vi "IsLogStopTriggered.vi"(7 "Application Configuration":T3={"DUT"={"Count"=1, "Wirings"=[], "Names"=[]}, "Log"={"Start"={"Trigger Type"=enum."Immediate", "Timer (sec)"=0.0, "Digital IO Line"=0, "Digital IO Edge"=enum."Rising"}, "Rollover"={"Trigger Type"=enum."None", "Timer (sec)"=0.0, "File Size (MB)"=0, "Digital IO Line"=0, "Digital IO Edge"=enum."Rising"}, "Stop"={"Trigger Type"=enum."None", "Timer (sec)"=0.0, "File Size (MB)"=0, "Digital IO Line"=0, "Digital IO Edge"=enum."Rising"}}, "Trigger"={"Input"={"Type"=enum."None", "Timeout (ms)"=0, "Delay (ms)"=0, "Digital IO Line (1-14)"=0, "Digital IO Mode"=enum."Falling"}, "Output"={"Type"=enum."None", "Delay (ms)"=0, "Digital IO Line (1-14)"=0, "Digital IO Mode"=enum."Falling", "Digital IO Pulse Width (sec)"=0.0}}, "Sources"=[], "Measures"=[]} {"Measures"."Count" min=1 step=1; "Trigger"."Output"."Digital IO Line (1-14)" min=1 max=14 step=1}, 8 "Error In":errorcluster, 11 "Log Data":T1[](array[typedef])) -> (0 "Error Out":errorcluster, 3 "Triggered?":bool)   [LabVIEW 2013]
uses:
  Setup.ctl
  DUTConfiguration.ctl
  driver/Public/Controls/SMUSense.ctl
  LogConfiguration.ctl
  LogStartConfiguration.ctl
  LogStartTriggerType.ctl
  LogDigitalIOTriggerEdge.ctl
  LogRolloverConfiguration.ctl
  LogRolloverTriggerType.ctl
  LogStopConfiguration.ctl
  LogStopTriggerType.ctl
  TriggerConfiguration.ctl
  TriggerInputConfiguration.ctl
  TriggerInputType.ctl
  driver/Public/Controls/TriggerMode.ctl
  TriggerOutputConfiguration.ctl
  TriggerOutputType.ctl
  SourceConfiguration.ctl
  SourceFunction.ctl
  MeasureConfiguration.ctl
  HardwareLogData.ctl
  HardwareDisplayData.ctl
  driver/Keithley-2602.lvlib
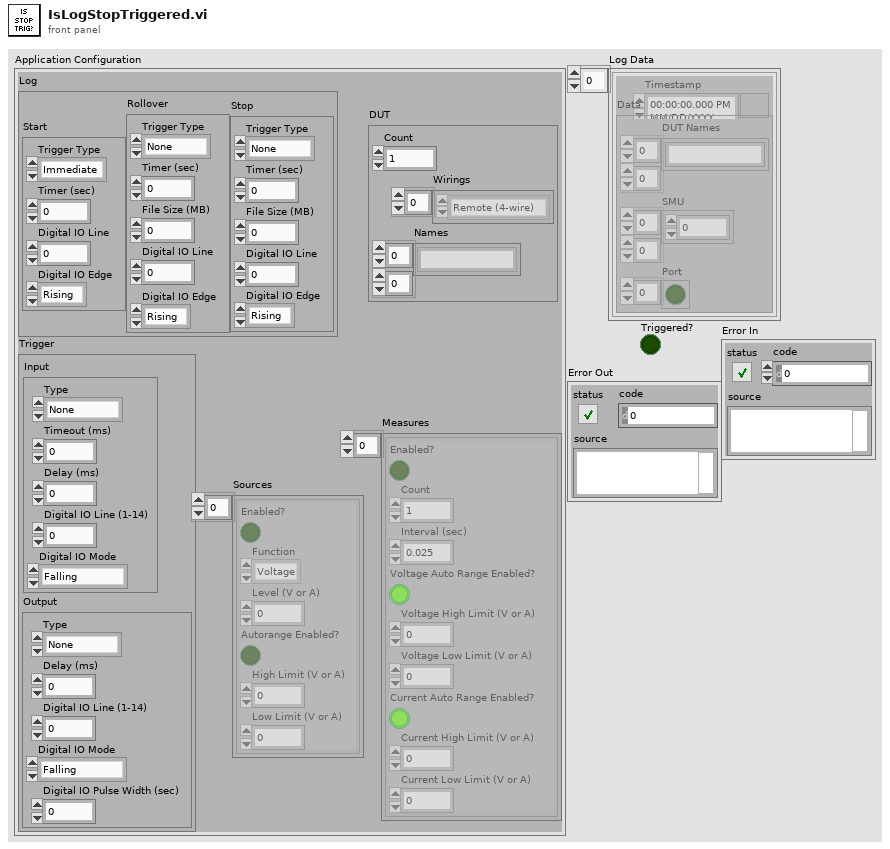
[diagram p1: front panel]
types:
  T1 = typedef "HardwareLogData.ctl" = cluster{"Timestamp":timestamp, "Data":T2}
  T2 = typedef "HardwareDisplayData.ctl" = cluster{"DUT Names":string[][], "SMU":dbl[][], "Port":bool[]}
  T3 = typedef "Setup.ctl" = cluster{"DUT":T4, "Log":T6, "Trigger":T14, "Sources":T20[], "Measures":T22[]}
  T4 = typedef "DUTConfiguration.ctl" = cluster{"Count":u32, "Wirings":T5[], "Names":string[][]}
  T5 = typedef "Keithley-2602.lvlib/SMUSense.ctl" = enum16{"Local (2-wire)", "Remote (4-wire)", "Calibration"}
  T6 = typedef "LogConfiguration.ctl" = cluster{"Start":T7, "Rollover":T10, "Stop":T12}
  T7 = typedef "LogStartConfiguration.ctl" = cluster{"Trigger Type":T8, "Timer (sec)":dbl, "Digital IO Line":u8, "Digital IO Edge":T9}
  T8 = typedef "LogStartTriggerType.ctl" = enum16{"Immediate", "User", "Timer", "Digital IO"}
  T9 = typedef "LogDigitalIOTriggerEdge.ctl" = enum16{"Rising", "Falling"}
  T10 = typedef "LogRolloverConfiguration.ctl" = cluster{"Trigger Type":T11, "Timer (sec)":dbl, "File Size (MB)":u32, "Digital IO Line":u8, "Digital IO Edge":T9}
  T11 = typedef "LogRolloverTriggerType.ctl" = enum16{"None", "Timer", "File Size", "Digital IO"}
  T12 = typedef "LogStopConfiguration.ctl" = cluster{"Trigger Type":T13, "Timer (sec)":dbl, "File Size (MB)":u32, "Digital IO Line":u8, "Digital IO Edge":T9}
  T13 = typedef "LogStopTriggerType.ctl" = enum16{"None", "User", "Timer", "File Size", "Digital IO"}
  T14 = typedef "TriggerConfiguration.ctl" = cluster{"Input":T15, "Output":T18}
  T15 = typedef "TriggerInputConfiguration.ctl" = cluster{"Type":T16, "Timeout (ms)":u32, "Delay (ms)":u32, "Digital IO Line (1-14)":u8, "Digital IO Mode":T17}
  T16 = typedef "TriggerInputType.ctl" = enum16{"None", "Digital IO", "Bus"}
  T17 = typedef "Keithley-2602.lvlib/TriggerMode.ctl" = enum16{"Falling", "Rising", "Either", "Synchronous"}
  T18 = typedef "TriggerOutputConfiguration.ctl" = cluster{"Type":T19, "Delay (ms)":u32, "Digital IO Line (1-14)":u8, "Digital IO Mode":T17, "Digital IO Pulse Width (sec)":dbl}
  T19 = typedef "TriggerOutputType.ctl" = enum16{"None", "Digital IO", "Bus"}
  T20 = typedef "SourceConfiguration.ctl" = cluster{"Enabled?":bool, "Function":T21, "Level (V or A)":dbl, "Autorange Enabled?":bool, "High Limit (V or A)":dbl, "Low Limit (V or A)":dbl}
  T21 = typedef "SourceFunction.ctl" = enum16{"Voltage", "Current"}
  T22 = typedef "MeasureConfiguration.ctl" = cluster{"Enabled?":bool, "Count":u8, "Interval (sec)":dbl, "Voltage Auto Range Enabled?":bool, "Voltage High Limit (V or A)":dbl, "Voltage Low Limit (V or A)":dbl, "Current Auto Range Enabled?":bool, "Current High Limit (V or A)":dbl, "Current Low Limit (V or A)":dbl}
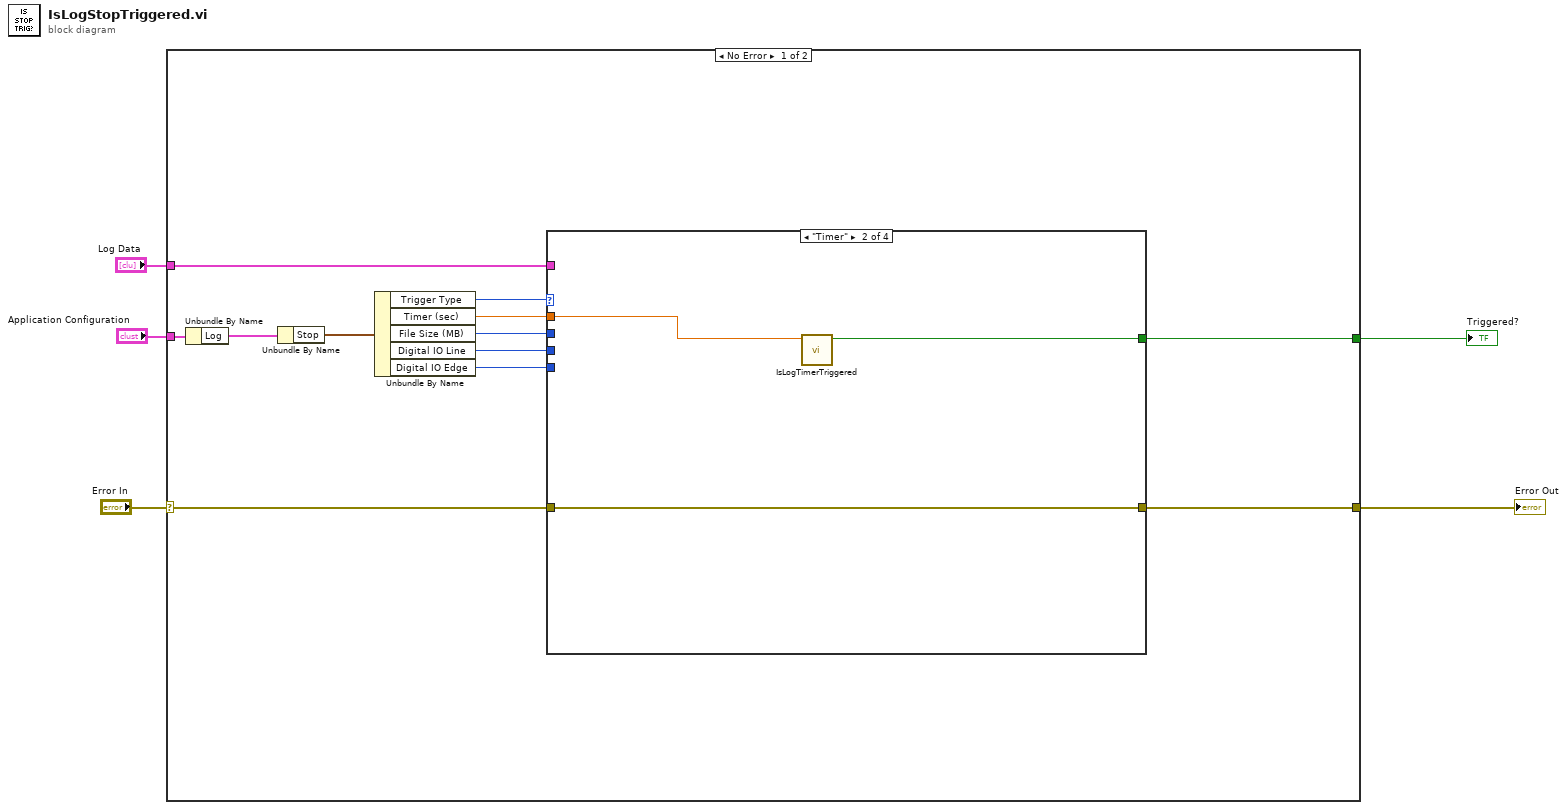
[diagram p0: block diagram]
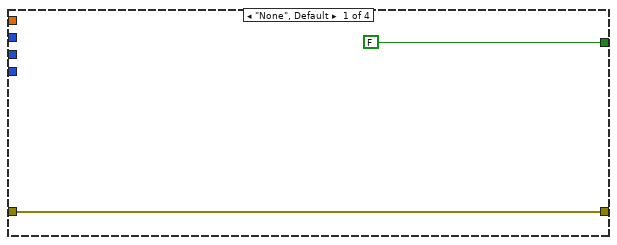
[diagram p2: hidden frame]
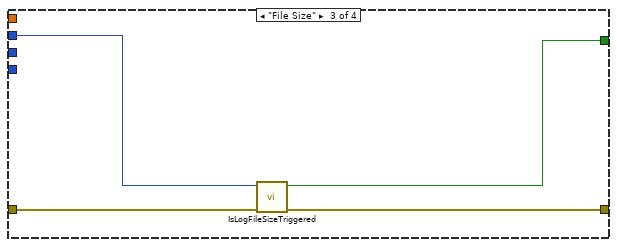
[diagram p3: hidden frame]
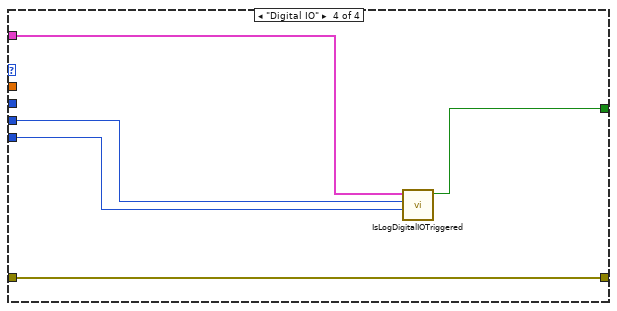
[diagram p4: hidden frame]
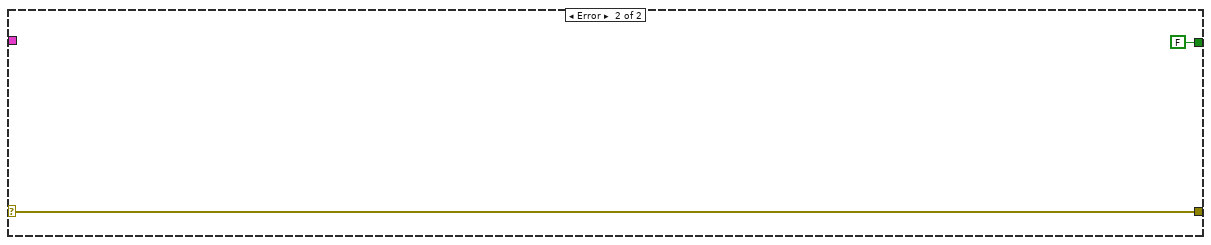
[diagram p5: hidden frame]
diagram:
  n1 = case shown="No Error" "Error In" {
    selector: "Error In" -> [w7 w33]
    tunnel: "Application Configuration" -> [w17 _]
    tunnel: [w9 w33] -> w4
    tunnel: [w8 FALSE ("Rollover?")] -> w3
    tunnel: "Log Data" -> [w6 _]
    frame No Error {
      n2 = Unbundle By Name(w17) -> ("Log"=w16:T6)
      n3 = Unbundle By Name(w16) -> ("Stop"=w15:T12)
      n4 = Unbundle By Name(w15) -> ("Trigger Type"=w14:T13, "Timer (sec)"=w13:dbl, "File Size (MB)"=w12:u32, "Digital IO Line"=w11:u8, "Digital IO Edge"=w10:T9)
      n5 = case shown="\"Timer\"" w14 {
        tunnel: [FALSE w20 w24 w31] -> w8
        tunnel: w13 -> [_ w21 _ _]
        tunnel: w12 -> [_ _ w23 _]
        tunnel: w11 -> [_ _ _ w29]
        tunnel: w10 -> [_ _ _ w28]
        tunnel: w6 -> [_ _ _ w30]
        tunnel: [w18 w22 w26 w27] -> w9
        tunnel: w7 -> [w18 w22 w25 w27]
        frame "None", Default {
        }
        frame "Timer" {
          n6 = call "IsLogTimerTriggered.vi"("Timer (sec)"=w21) -> ("Triggered?"=w20:bool)  [unwired: 10 in]
        }
        frame "File Size" {
          n7 = call "IsLogFileSizeTriggered.vi"("Error In"=w25, "File Size (MB)"=w23) -> ("Error Out"=w26:errorcluster, "Triggered?"=w24:bool)  [unwired: 8 in]
        }
        frame "Digital IO" {
          n8 = call "IsLogDigitalIOTriggered.vi"("Digital IO Edge"=w28, "Digital IO Line"=w29, "Log Data"=w30) -> ("Triggered?"=w31:bool)  [unwired: 8 in]
        }
      }
    }
    frame Error {
    }
  }
  "Error Out" <- w4
  "Triggered?" <- w3
